vi "lab_3_partie_4_C.vi"() -> ()   [LabVIEW 2020]
uses:
  <instrlib>/Agilent E363X Series/Agilent E363X Series.lvlib
panel:
  in  "Incrément tension base":dbl step=0.05
  in  "Tension base max":dbl
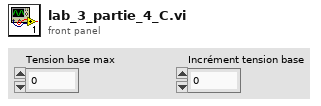
[diagram p1: front panel]
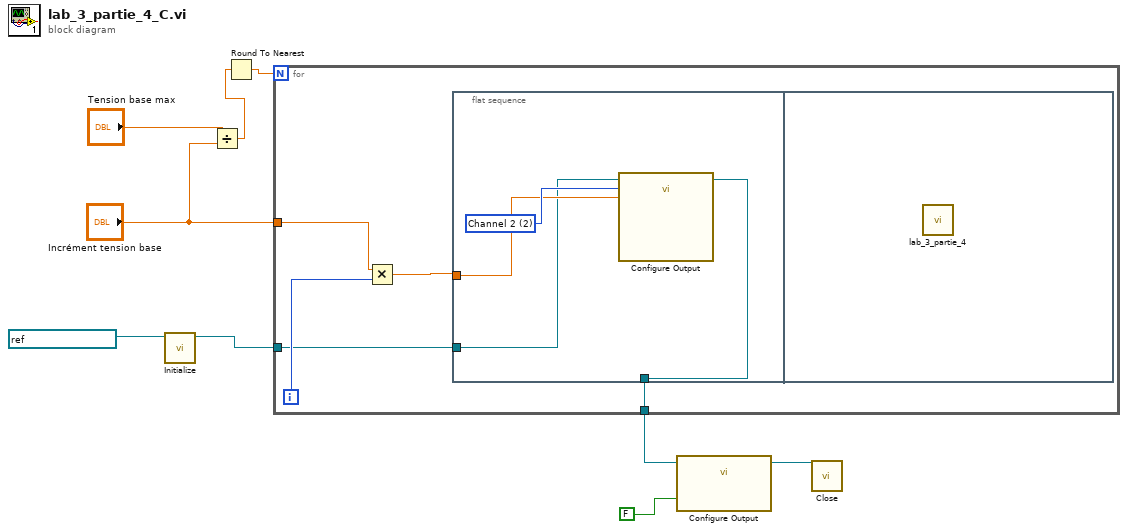
[diagram p0: block diagram]
diagram:
  n1 = call <instrlib>:"Initialize.vi"("VISA resource name"=refnum<visa-resource-name> "GPIB0::5::INSTR") -> ("VISA resource name out"=w5:refnum<visa-resource-name>)  [unwired: 9 in, 1 out]
  n2 = Divide(x="Tension base max", y="Incrément tension base") -> (x/y=w7:dbl)
  n3 = Round To Nearest(number=w7) -> (nearest integer value=w6:dbl)
  n4 = for {
    N: w6 -> [_]
    tunnel: "Incrément tension base" -> [w12]
    tunnel: w5 -> [w11]
    tunnel: [w10] -> w3
    i -> [w13]
    n5 = Multiply(x=w12, y=w13) -> (x*y=w14:dbl)
    n6 = flat-sequence {
      tunnel: w14 -> [w17]
      tunnel: w11 -> [w16]
      tunnel: [w15] -> w10
      frame #0 {
        w18 = 2 items=["Channel 1"=1, "Channel 2"=2, "Channel 3"=3] ("Channel (1: Channel 1)")
        n7 = call <instrlib>:"Configure Output.vi"("Voltage Level (0.0 V)"=w17, "Channel (1: Channel 1)"=w18, "VISA resource name"=w16) -> ("VISA resource name out"=w15:refnum<visa-resource-name>)  [unwired: 7 in, 1 out]
      }
      frame #1 {
        n8 = call "lab_3_partie_4.vi"() -> ()  [unwired: 12 in]
      }
    }
  }
  n9 = call <instrlib>:"Configure Output.vi"("Enable Output (T: Enable)"=FALSE, "VISA resource name"=w3) -> ("VISA resource name out"=w2:refnum<visa-resource-name>)  [unwired: 8 in, 1 out]
  n10 = call <instrlib>:"Close.vi"("VISA resource name"=w2) -> ()  [unwired: 10 in, 1 out]
